vi "verify expouse time.vi"(8 "error in (no error)":errorcluster, 11 "Simulated_CCD_Camera in":refnum<class "Simulated Camera.lvclass">) -> (0 "error out":errorcluster, 3 "Simulated_CCD_Camera out":refnum<class "Simulated Camera.lvclass">)   [LabVIEW 2018, in "Simulated Camera.lvclass"]
uses:
  Simulated Camera.lvclass
  Simulated Camera.lvclass/Simulated Camera.ctl
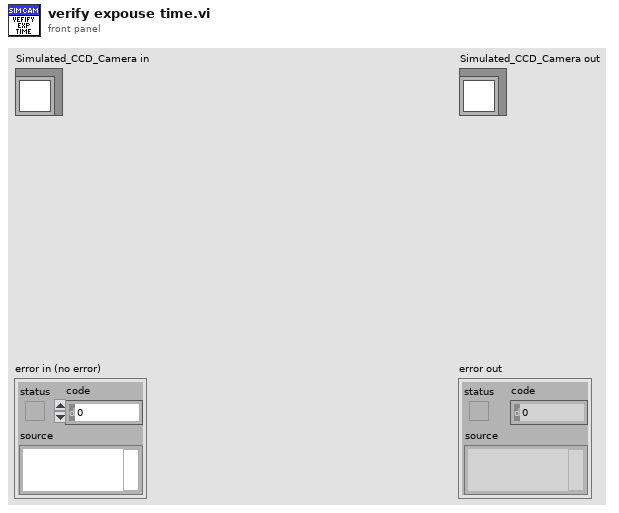
[diagram p1: front panel]
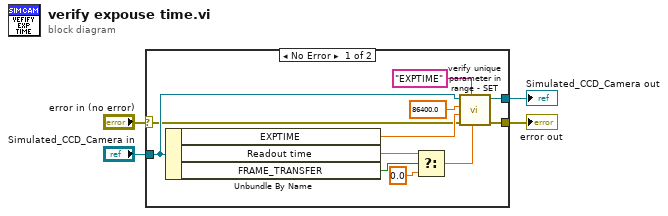
[diagram p0: block diagram]
diagram:
  n1 = case shown="No Error" "error in (no error)" {
    selector: "error in (no error)" -> [w5 w17]
    tunnel: [w8 w17] -> w3
    tunnel: [w7 w16] -> w1
    tunnel: "Simulated_CCD_Camera in" -> [w6 w16]
    frame No Error {
      n2 = Unbundle By Name(w6) -> ("EXPTIME"=w10:dbl, "Readout time"=w14:dbl, "FRAME_TRANSFER"=w15:bool)
      n3 = Select(t=w14, s=w15, f=0.0) -> (s? t:f=w9:dbl)
      n4 = call "verify unique parameter in range - SET.vi"("lower limit"=w9, "parameter name"="EXPTIME", "error in (no error)"=w5, "value"=w10, "upper limit"=86400.0, "Simulated_CCD_Camera in"=w6) -> ("error out"=w8:errorcluster, "Simulated_CCD_Camera out"=w7:refnum<class "Simulated Camera.lvclass">)  [unwired: 4 in]
    }
    frame Error {
    }
  }
  "error out" <- w3
  "Simulated_CCD_Camera out" <- w1
